vi "global-velocity-graph.vi"() -> ()   [LabVIEW 2020]
uses:
  Global-velocity.vi
panel:
  out "Waveform Graph":dbl[](graph)
  in  "stop":bool
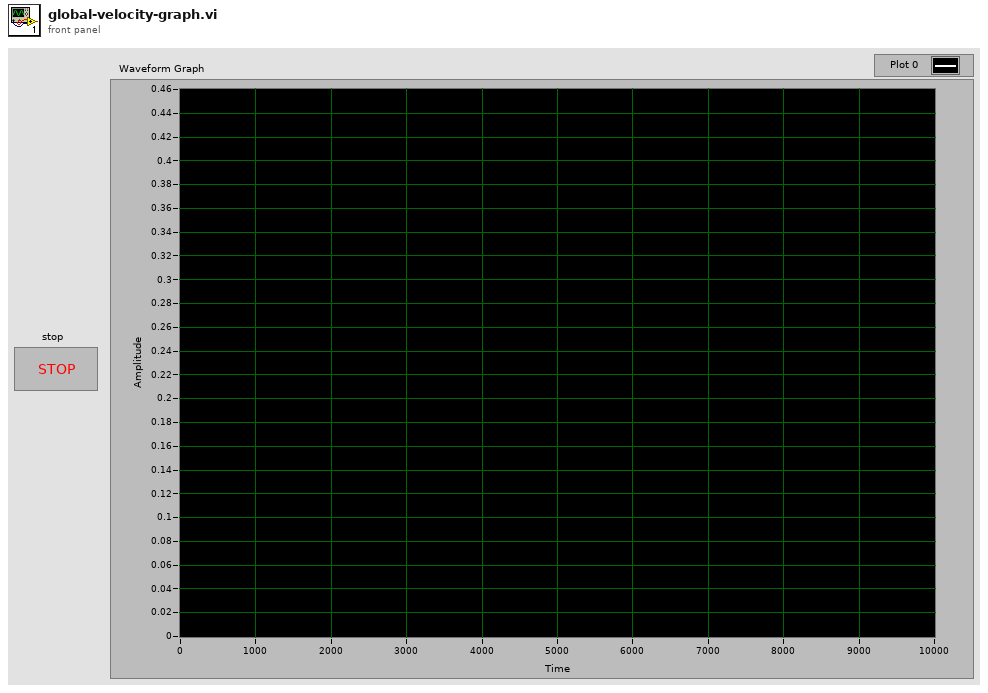
[diagram p1: front panel]
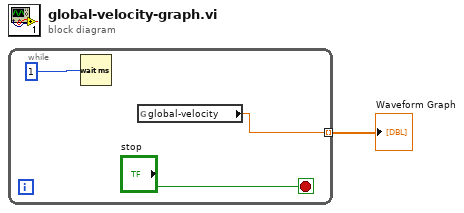
[diagram p0: block diagram]
diagram:
  n1 = while {
    tunnel: [w2] -> w1 mode=indexing
    stop <- "stop" stop-if-true
    n2 = Wait (ms)(milliseconds to wait=1) -> ()  [unwired: 1 out]
    n3 = global read "Global-velocity.vi" "global-velocity"() -> (w2:dbl)
  }
  "Waveform Graph" <- w1
